vi "SQLite Update Template.vi"(7 "PK":cluster{}, 8 "error in":errorcluster, 9 "Fields":string[](array[combo]), 10 "Data":cluster{}, 11 "SQLite Connection in":refnum<class "Connection.lvclass">) -> (0 "error out":errorcluster, 3 "SQLite Connection out":refnum<class "Connection.lvclass">)   [LabVIEW 2021]
uses:
  <vilib>/drjdpowell/SQLite Library/SQL Connection/Connection.lvclass
  <vilib>/drjdpowell/SQLite Library/SQL Statement/SQL Statement.lvclass
  <vilib>/drjdpowell/SQLite Library/Transaction Helpers/Transaction.lvlib
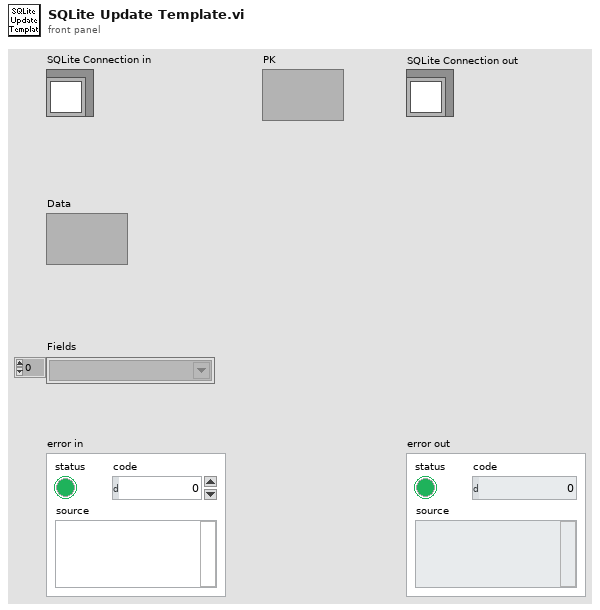
[diagram p1: front panel]
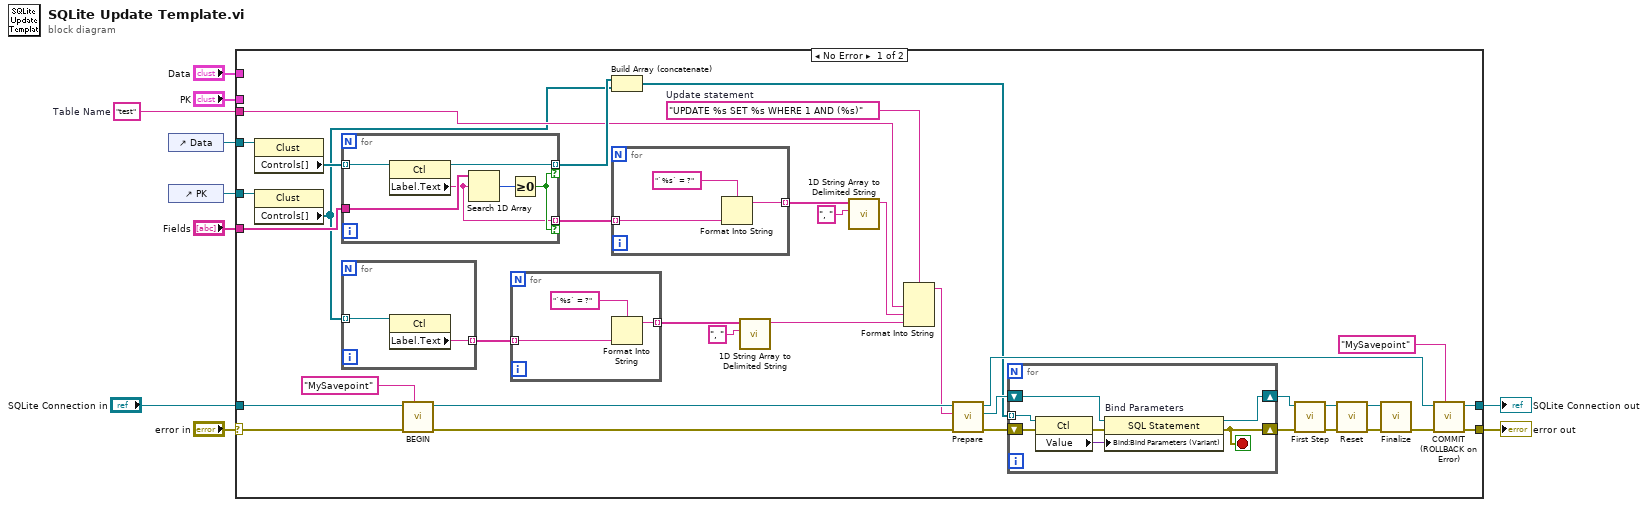
[diagram p0: block diagram]
diagram:
  w6 = "test"  # Table Name
  n1 = control-ref of="Data"() -> (w4:refnum<vi>)
  n2 = control-ref of="PK"() -> (w1:refnum<vi>)
  n3 = case shown="No Error" "error in" {
    selector: "error in" -> [w39 w69]
    tunnel: [w37 w69] -> w9
    tunnel: "SQLite Connection in" -> [w38 w68]
    tunnel: [w36 w68] -> w7
    tunnel: w6 -> [w19 _]
    tunnel: "Data" -> [_ _]
    tunnel: w4 -> [w33 _]
    tunnel: "Fields" -> [w27 _]
    tunnel: "PK" -> [_ _]
    tunnel: w1 -> [w26 _]
    frame No Error {
      w21 = "UPDATE %s SET %s WHERE 1 AND (%s)"  # Update statement
      n4 = property class="Clust"(reference=w33) -> ("Controls[]"=w32:refnum<vi>[])  [unwired: 1 in, 2 out]
      n5 = property class="Clust"(reference=w26) -> ("Controls[]"=w15:refnum<vi>[])  [unwired: 1 in, 2 out]
      n6 = for {
        tunnel: w32 -> [w67] mode=indexing
        tunnel: w27 -> [w65]
        tunnel: [w66] -> w24 mode=indexing if=w63
        tunnel: [w62] -> w17 mode=indexing if=w63
        n7 = property class="Ctl"(reference=w67) -> (reference out=w66:refnum<vi>, "Label.Text"=w62:string)  [unwired: 1 in, 1 out]
        n8 = Search 1D Array(1D array=w65, element=w62) -> (index of element=w64:i32)  [unwired: 1 in]
        n9 = Greater Or Equal To 0?(x=w64) -> (x >= 0?=w63:bool)
      }
      n10 = for {
        tunnel: w15 -> [w61] mode=indexing
        tunnel: [w60] -> w14 mode=indexing
        n11 = property class="Ctl"(reference=w61) -> ("Label.Text"=w60:string)  [unwired: 1 in, 2 out]
      }
      n12 = call <vilib>:"BEGIN.vi"("Savepoint name"="MySavepoint", "error in (no error)"=w39, "SQLite Connection in"=w38) -> ("error out"=w42:errorcluster, "SQLite Connection"=w43:refnum<class "Connection.lvclass">)  [unwired: 7 in]
      n13 = for {
        tunnel: w14 -> [w55] mode=indexing
        tunnel: [w54] -> w12 mode=indexing
        n14 = Format Into String(format string="`%s` = ?", w55) -> (resulting string=w54:string)  [unwired: 2 in, 1 out]
      }
      n15 = Build Array (concatenate)(w24, w15) -> (w16:refnum<vi>[])
      n16 = for {
        tunnel: w17 -> [w58] mode=indexing
        tunnel: [w57] -> w20 mode=indexing
        n17 = Format Into String(format string="`%s` = ?", w58) -> (resulting string=w57:string)  [unwired: 2 in, 1 out]
      }
      n18 = call <vilib>:"1D String Array to Delimited String.vi"("delimiter"=", ", "string array"=w12) -> ("delimited string"=w11:string)  [unwired: 9 in]
      n19 = call <vilib>:"1D String Array to Delimited String.vi"("delimiter"=", ", "string array"=w20) -> ("delimited string"=w23:string)  [unwired: 9 in]
      n20 = Format Into String(format string=w21, w19, w23, w11) -> (resulting string=w18:string)  [unwired: 2 in, 1 out]
      n21 = call <vilib>:"Prepare.vi"("error in (no error)"=w42, "SQL"=w18, "SQLite Connection in"=w43) -> ("error out"=w46:errorcluster, "SQL Statement"=w25:refnum<class "SQL Statement.lvclass">, "SQLite Connection"=w41:refnum<class "Connection.lvclass">)  [unwired: 4 in, 2 out]
      n22 = for {
        tunnel: w16 -> [w51] mode=indexing
        shift-right: [w52] -> w31
        shift-left: w25 -> [w50]
        shift-right: [w48] -> w30
        shift-left: w46 -> [w49]
        stop <- w48 stop-if-true
        n23 = property class="Ctl"(reference=w51, error in=w49) -> (error out=w53:errorcluster, "Value"=w47:variant)  [unwired: 1 out]
        n24 = property on="Bind Parameters" class="SQL Statement"(reference=w50, error in=w53, "Bind:Bind Parameters (Variant)"=w47) -> (reference out=w52:refnum<class "SQL Statement.lvclass">, error out=w48:errorcluster)
      }
      n25 = call <vilib>:"First Step.vi"("error in (no error)"=w30, "SQL Statement in"=w31) -> ("error out"=w29:errorcluster, "SQL Statement"=w28:refnum<class "SQL Statement.lvclass">)  [unwired: 7 in, 1 out]
      n26 = call <vilib>:"Reset.vi"("error in (no error)"=w29, "SQL Statement in"=w28) -> ("error out"=w44:errorcluster, "SQL Statement"=w45:refnum<class "SQL Statement.lvclass">)  [unwired: 8 in]
      n27 = call <vilib>:"Finalize.vi"("error in (no error)"=w44, "SQL Statement in"=w45) -> ("error out"=w40:errorcluster)  [unwired: 9 in]
      n28 = call <vilib>:"COMMIT (ROLLBACK on Error).vi"("Savepoint name"="MySavepoint", "error in (no error)"=w40, "SQLite Connection in"=w41) -> ("error out"=w37:errorcluster, "SQLite Connection"=w36:refnum<class "Connection.lvclass">)  [unwired: 7 in]
    }
    frame Error {
    }
  }
  "error out" <- w9
  "SQLite Connection out" <- w7
